vi "WVD Spectrogram PtByPt.vi"(0 "x":dbl format="%0.2f", 1 "sample length":i32=100, 3 "time increment":i32=100, 4 "initialize":bool) -> (5 "WVD Spectrogram {X}":dbl[][](array[numeric]), 6 "error":i32)   [LabVIEW 2020, in "NI_PtbyPt.lvlib"]
doc: "Computes the signal energy distribution in the joint time-frequency domain using the Wigner-Ville distribution algorithm."
uses:
  <vilib>/ptbypt/NI_PtbyPt.lvlib
  <vilib>/gmath/NI_Gmath.lvlib
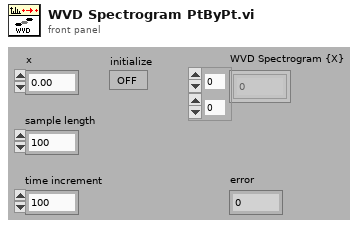
[diagram p1: front panel]
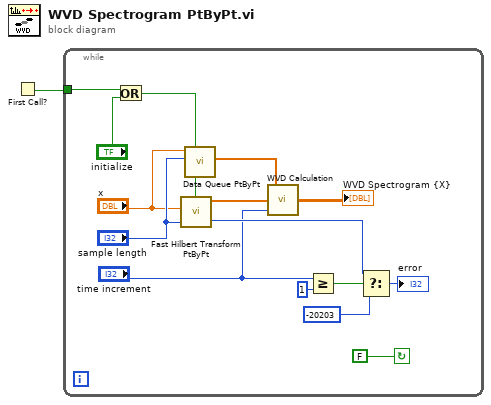
[diagram p0: block diagram]
diagram:
  n1 = First Call?() -> (First Call?: T/F=w1:bool)
  n2 = while {
    tunnel: w1 -> [w4]
    stop <- FALSE continue-if-true
    n3 = Or(x=w4, y="initialize") -> (x .or. y?=w5:bool)
    n4 = call <vilib>:"Fast Hilbert Transform PtByPt.vi"("initialize"=w5, "sample length"="sample length", "x"="x") -> ("error"=w8:i32, "Hilbert{X}"=w15:dbl[])  [unwired: 1 in]
    n5 = call <vilib>:"Data Queue PtByPt.vi"("initialize"=w5, "sample length"="sample length", "input data point"="x") -> ("Current Queue"=w13:dbl[])  [unwired: 4 in, 4 out]
    n6 = call <vilib>:"WVD Calculation.vi"("time increment"="time increment", "H[s]"=w15, "s"=w13) -> ("Fourier[s(i-m)*g(m)]"=→"WVD Spectrogram {X}":sgl[][])
    n7 = Greater Or Equal?(x="time increment", y=1) -> (x >= y?=w11:bool)
    n8 = Select(t=w8, s=w11, f=-20203) -> (s? t:f=→"error":i32)
  }
